vi "PCO_GetFlimPhaseSequenceParameter.vi"(0 "ph":u64, 11 "error in (no error)":errorcluster {"code" format="%x"}) -> (3 "wPhaseOrder":u16(ring) items=["ascending", "opposite"], 4 "ph out":u64, 6 "ErrorMessage":i32 format="%x", 8 "wPhaseNumber":u16(ring) items=["shiftablePair", "2", "4", "8", "16"], 10 "wPhaseSymmetry":u16(ring) items=["no", "yes"], 14 "wTapSelect":u16(ring) items=["Tap A+B", "Tap A", "Tap B"], 15 "error out":errorcluster {"code" format="%x"})   [LabVIEW 2020, in "SDK.lvlib" / "SpecialCommandsFlim.lvlib"]
doc: "<b>Description:</b>\nGet configuration for the generation of phase image sequences. The combination of the described options determines the resulting length and sorting of phase sequences. One phase sequence is a sequence of single (phase) images sampled at different points within the full modulation period of 360°. Because each parameter has an influence on each other, table Image Sequences should be used to determine the resulting image sequence.\n\n<b>Supported camera type:</b>\npco.flim\n\n<b>Descriptor dependency:</b>\nNone"
uses:
  SpecialCommandsFlim.lvlib
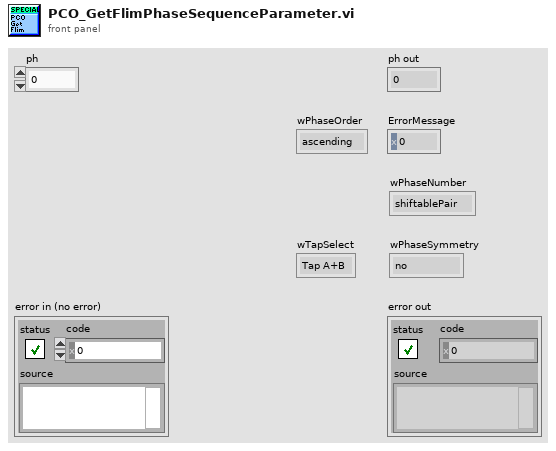
[diagram p1: front panel]
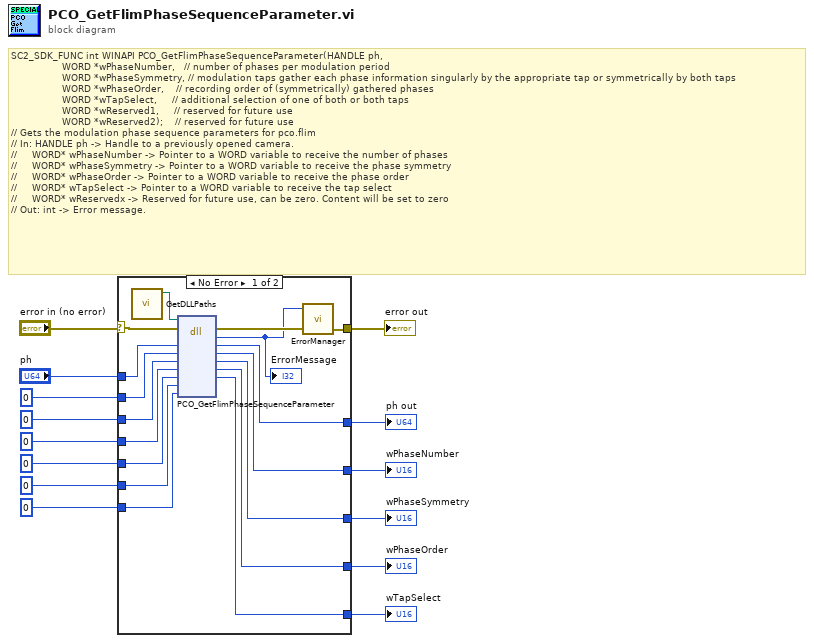
[diagram p0: block diagram]
diagram:
  # "SC2_SDK_FUNC int WINAPI PCO_GetFlimPhaseSequenceParameter(HANDLE ph, \n                 WORD *wPhaseNumber,   // number of phases per modulation period\n                 WORD *wPhaseSymmetry, // modulation taps gather each phase information singularly by the appropriate tap or symmetrically by both taps\n                 WORD *wPhaseOrder,    // recording order of (symmetrically) gathered phases\n                 WORD *wTapSelect,     // additional selection of one of both or both taps\n                 WORD *wReserved1,     // reserved for future use\n                 WORD *wReserved2);    // reserved for future use\n// Gets the modulation phase sequence parameters for pco.flim\n// In: HANDLE ph -> Handle to a previously opened camera.\n//     WORD* wPhaseNumber -> Pointer to a WORD variable to receive the number of phases\n//     WORD* wPhaseSymmetry -> Pointer to a WORD variable to receive the phase symmetry\n//     WORD* wPhaseOrder -> Pointer to a WORD variable to receive the phase order\n//     WORD* wTapSelect -> Pointer to a WORD variable to receive the tap select\n//     WORD* wReservedx -> Reserved for future use, can be zero. Content will be set to zero\n// Out: int -> Error message."
  n1 = case shown="No Error" "error in (no error)" {
    selector: "error in (no error)" -> [w19 w37]
    tunnel: "ph" -> [w31 w36]
    tunnel: [w30 w36] -> w13
    tunnel: u16 0 ("wPhaseNumber") -> [w29 w35]
    tunnel: [w28 w35] -> w11
    tunnel: u16 0 ("wPhaseSymmetry") -> [w27 w34]
    tunnel: [w26 w34] -> w9
    tunnel: u16 0 ("wPhaseOrder") -> [w25 w33]
    tunnel: [w24 w33] -> w7
    tunnel: u16 0 ("wTapSelect") -> [w23 w32]
    tunnel: [w22 w32] -> w5
    tunnel: u16 0 ("wReserved1") -> [w21 _]
    tunnel: u16 0 ("wReserved2") -> [w20 _]
    tunnel: [w18 w37] -> w2
    frame No Error {
      n2 = call "GetDLLPaths.vi"() -> ("SC2_Cam_Path"=w15:path)  [unwired: 9 in, 2 out]
      n3 = dll-call lib="?" fn="PCO_GetFlimPhaseSequenceParameter"(path in=w15, error in=w19, "ph"=w31, "wPhaseNumber"=w29, "wPhaseSymmetry"=w27, "wPhaseOrder"=w25, "wTapSelect"=w23, "wReserved1"=w21, "wReserved2"=w20) -> (error out=w17:errorcluster, "return type"=w16:i32, "ph"=w30:u64, "wPhaseNumber"=w28:u16, "wPhaseSymmetry"=w26:u16, "wPhaseOrder"=w24:u16, "wTapSelect"=w22:u16)  [unwired: 3 in, 1 out]
      "ErrorMessage" <- w16
      n4 = call "ErrorManager.vi"("error in (no error)"=w17, "error code"=w16) -> ("error out"=w18:errorcluster)  [unwired: 3 in]
    }
    frame Error {
    }
  }
  "ph out" <- w13
  "wPhaseNumber" <- w11
  "wPhaseSymmetry" <- w9
  "wPhaseOrder" <- w7
  "wTapSelect" <- w5
  "error out" <- w2
